vi "Autonomous Independent.vi"   [LabVIEW 2023]
doc: "This VI is called when autonomous begins, and will automatically be terminated when autonomous ends. You can carry out timed or sensor driven robot movement independently without needing to return to the caller."
uses:
  <vilib>/Rock Robotics/WPI/Utilities/WPI_GetSetVariantRefNum.vi
  <vilib>/Rock Robotics/WPI/RobotDrive/WPI_RobotDriveMecanumDrive_Cartesian.vi
  <vilib>/Rock Robotics/Network Tables/NT Read Number.vi
  <vilib>/Rock Robotics/Network Tables/NT Read String.vi
panel:
  # "Be sure to right-click and choose Data Operations>>Make Current Value default if you want to save the array values with the VI"
types:
  T1 = typedef "WPI_RobotDriveDevRef.ctl" = cluster{"DevStatus":errorcluster, "Motors[]":T2[], "Square Inputs":bool, "Max Output":dbl}
  T2 = typedef "WPI_MotorControlDeviceRef.ctl" = cluster{"DeviceStatus":errorcluster, "Type":T3, "PWM":cluster{"PWM Channel":T4, "DeadBand":T5}, "CAN":cluster{"Device Number":u8, "SetOutput VI Ref":variant, "GetOutput VI Ref":variant, "Enable VI Ref":variant, "Disable VI Ref":variant, "Data":variant}, "Invert":bool, "DIO PWM":cluster{"PWM \"Enable\" Channel":T4, "DIOChannel":T6, "PWM Rate":dbl}}
  T3 = typedef "WPI_MotorControlType.ctl" = enum16{"PWM", "CAN", "DIO PWM"}
  T4 = typedef "FPGA_DIOPWMChannel.ctl" = enum8{"PWM 0", "PWM 1", "PWM 2", "PWM 3", "PWM 4", "PWM 5", "PWM 6", "PWM 7", "PWM 8", "PWM 9", "PWM MXP 0", "PWM MXP 1", "PWM MXP 2", "PWM MXP 3", "PWM MXP 4", "PWM MXP 5", "PWM MXP 6", "PWM MXP 7", "PWM MXP 8", "PWM MXP 9", "Invalid"}
  T5 = typedef "WPI_PWMDeadband.ctl" = cluster{"Name":string, "maxPositivePwm":i32, "minPositivePwm":i32, "centerPwm":i32, "maxNegativePwm":i32, "minNegativePwm":i32, "angularRange":u16}
  T6 = typedef "FPGA_DIOChannel.ctl" = enum8{"DIO 0", "DIO 1", "DIO 2", "DIO 3", "DIO 4", "DIO 5", "DIO 6", "DIO 7", "DIO 8", "DIO 9", "DIO MXP 0", "DIO MXP 1", "DIO MXP 2", "DIO MXP 3", "DIO MXP 4", "DIO MXP 5", "DIO MXP 6", "DIO MXP 7", "DIO MXP 8", "DIO MXP 9", "DIO MXP 10", "DIO MXP 11", "DIO MXP 12", "DIO MXP 13", "DIO MXP 14", "DIO MXP 15", "SPI Port CS1", "SPI Port CS2", "SPI Port CS3", "SPI Port MISO", "SPI Port MOSI", "Invalid"}
  T7 = typedef "WPI_GyroDevRef.ctl" = cluster{"DevStatus":errorcluster, "Analog Channel":T8, "Gain (VoltsPerDegree/Second)":dbl, "Gyro Type":enum16{"Analog", "XRS450"}, "Handle":i32, "SPI Bus":T9, "Device Found":bool, "Sample Rate":dbl, "Calibrate On Open":bool, "Offset":dbl}
  T8 = typedef "FPGA_AIChannel.ctl" = enum8{"AI 0", "AI 1", "AI 2", "AI 3", "AI MXP 0", "AI MXP 1", "AI MXP 2", "AI MXP 3", "Invalid"}
  T9 = typedef "spi_bus.ctl" = enum16{"SPI On-Board, CS0", "SPI On-Board, CS1", "SPI On-Board, CS2", "SPI On-Board, CS3", "SPI MXP", "Invalid"}
  T10 = typedef "WPI_DigitalInputDevRef.ctl" = cluster{"DevStatus":errorcluster, "DIO Channel":T6}
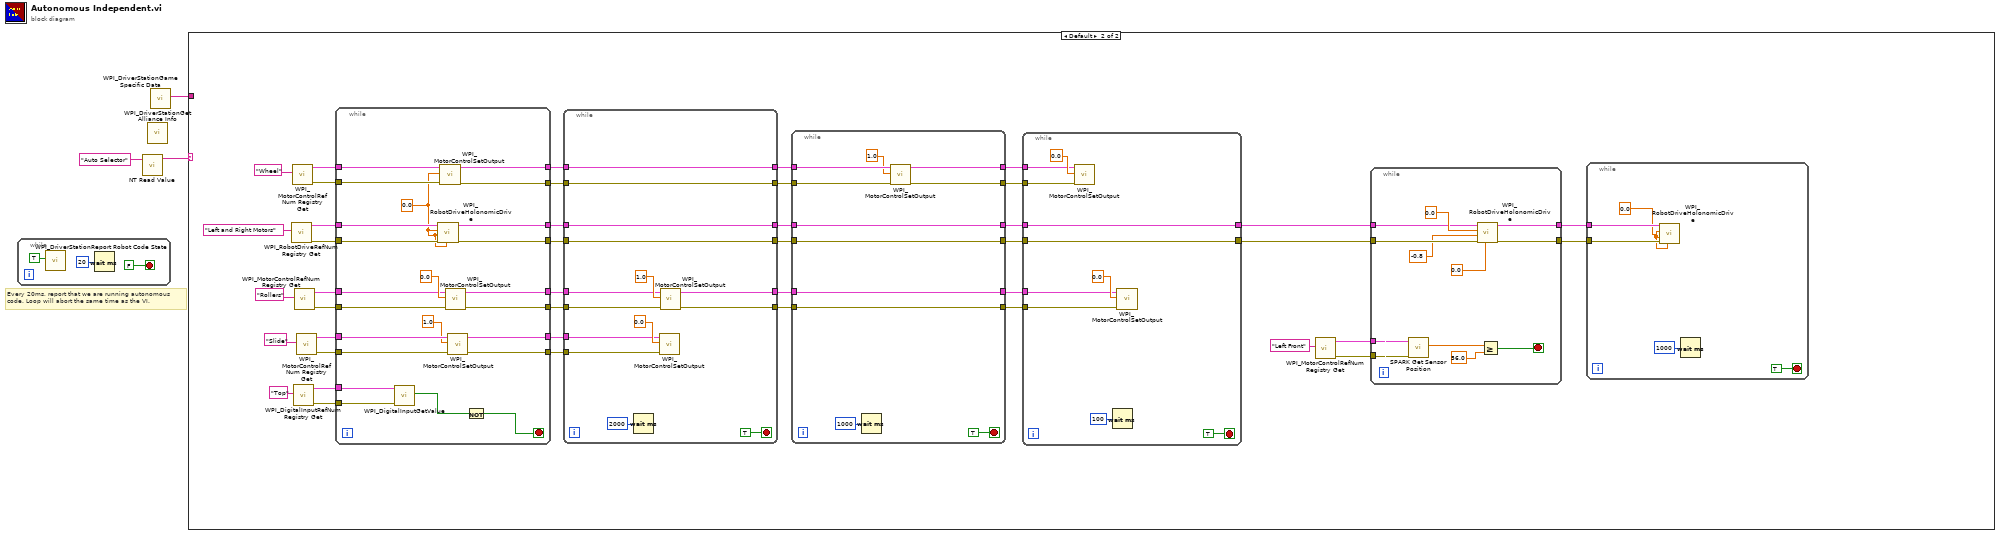
[diagram p0: block diagram]
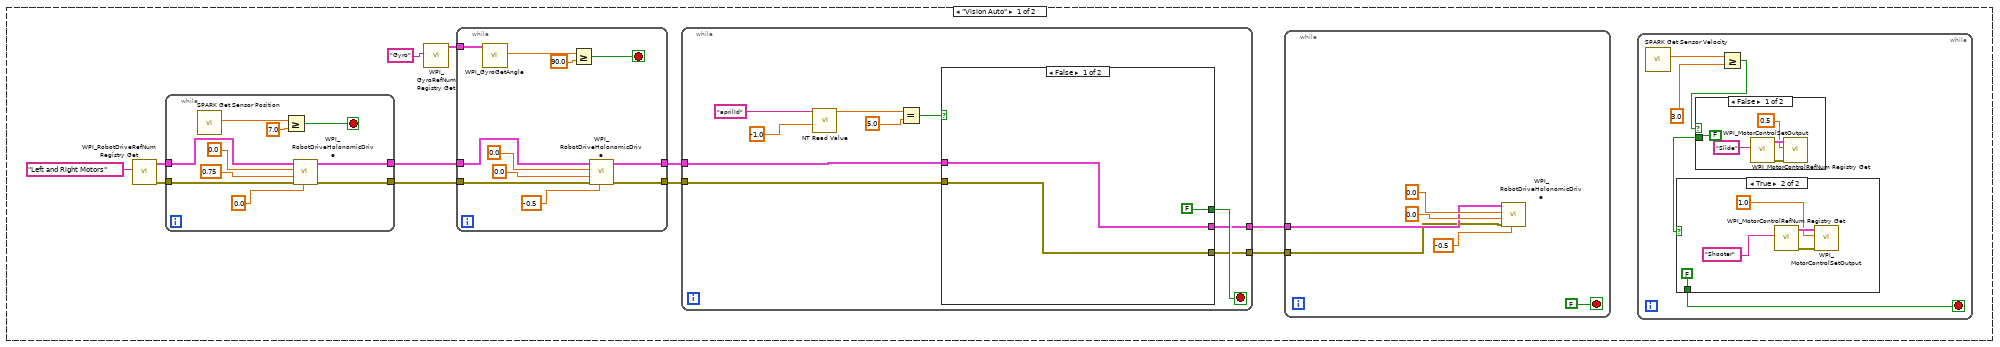
[diagram p2: hidden frame]
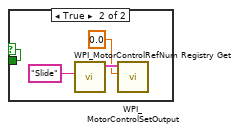
[diagram p3: hidden frame]
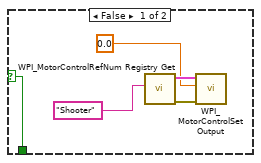
[diagram p4: hidden frame]
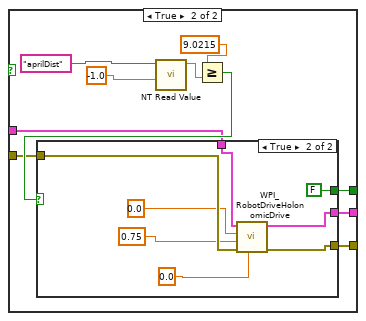
[diagram p5: hidden frame]
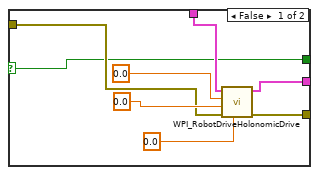
[diagram p6: hidden frame]
diagram:
  # "Every 20ms, report that we are running autonomous\ncode. Loop will abort the same time as the VI."
  n1 = while {
    stop <- FALSE stop-if-true
    n2 = call <vilib>:"WPI_DriverStationReport Robot Code State.vi"("Autonomous"=TRUE) -> ()  [unwired: 10 in, 1 out]
    n3 = Wait (ms)(milliseconds to wait=u32 20) -> ()  [unwired: 1 out]
  }
  n4 = call-poly <vilib>:"NT Read Value.vi"("name"="Auto Selector" ("Name")) -> ("value"=w2:string)  [unwired: 8 in, 2 out]
  n5 = call <vilib>:"WPI_DriverStationGet Alliance Info.vi"() -> ()  [unwired: 12 out]
  n6 = call <vilib>:"WPI_DriverStationGame Specific Data.vi"() -> ("Game Specific Data"=w1:string)  [unwired: 11 in]
  n7 = case shown="Default" w2 {
    tunnel: w1 -> [_ _]
    frame "Vision Auto" {
      n8 = call <vilib>:"WPI_RobotDriveRefNum Registry Get.vi"("refnum name"="Left and Right Motors") -> ("error out"=w16:errorcluster, "RobotDriveDevRef"=w15:T1)  [unwired: 1 in, 8 out]
      n9 = while {
        tunnel: w16 -> [w106]
        tunnel: w15 -> [w103]
        tunnel: [w99] -> w14
        tunnel: [w98] -> w13
        stop <- w100 stop-if-true
        n10 = call <vilib>:"SPARK Get Sensor Position.vi"() -> ("Sensor Position"=w102:dbl)  [unwired: 8 in, 3 out]
        n11 = Greater Or Equal?(x=w102, y=7.0) -> (x >= y?=w100:bool)
        n12 = call-poly <vilib>:"WPI_RobotDriveHolonomicDrive.vi"("Rotation"=0.0, "error in (no error)"=w106, "Y"=0.75, "X"=0.0, "RobotDriveDevRef"=w103) -> ("error out"=w98:errorcluster, "RobotDriveDevRef"=w99:T1)  [unwired: 4 in, 1 out]
      }
      n13 = call <vilib>:"WPI_GyroRefNum Registry Get.vi"("refnum name"="Gyro") -> ("GyroDevRef"=w11:T7)  [unwired: 9 in, 1 out]
      n14 = while {
        tunnel: w14 -> [w97]
        tunnel: w13 -> [w96]
        tunnel: w11 -> [w90]
        tunnel: [w88] -> w10
        tunnel: [w87] -> w9
        stop <- w89 stop-if-true
        n15 = call <vilib>:"WPI_GyroGetAngle.vi"("GyroDevRef"=w90) -> ("Angle"=w91:dbl)  [unwired: 6 in, 4 out]
        n16 = Greater Or Equal?(x=w91, y=90.0) -> (x >= y?=w89:bool)
        n17 = call-poly <vilib>:"WPI_RobotDriveHolonomicDrive.vi"("Rotation"=-0.5, "error in (no error)"=w96, "Y"=0.0, "X"=0.0, "RobotDriveDevRef"=w97) -> ("error out"=w87:errorcluster, "RobotDriveDevRef"=w88:T1)  [unwired: 4 in, 1 out]
      }
      n18 = while {
        tunnel: w10 -> [w51]
        tunnel: w9 -> [w52]
        tunnel: [w49] -> w8
        tunnel: [w48] -> w7
        stop <- w50 stop-if-true
        n19 = call-poly <vilib>:"NT Read Value.vi"("default value"=-1.0, "name"="aprilId") -> ("value"=w55:dbl)  [unwired: 7 in, 2 out]
        n20 = Equal?(x=w55, y=5.0) -> (x = y?=w53:bool)
        n21 = case shown="False" w53 {
          tunnel: w52 -> [w58 w65]
          tunnel: w51 -> [w59 w64]
          tunnel: [FALSE w63] -> w50
          tunnel: [w59 w62] -> w49
          tunnel: [w58 w61] -> w48
          frame False {
          }
          frame True {
            n22 = call-poly <vilib>:"NT Read Value.vi"("default value"=-1.0, "name"="aprilDist") -> ("value"=w70:dbl)  [unwired: 7 in, 2 out]
            n23 = Greater Or Equal?(x=9.0215, y=w70) -> (x >= y?=w66:bool)
            n24 = case shown="True" w66 {
              selector: w66 -> [w73 _]
              tunnel: w65 -> [w74 w85]
              tunnel: w64 -> [w75 w82]
              tunnel: [w73 FALSE] -> w63
              tunnel: [w72 w80] -> w62
              tunnel: [w71 w79] -> w61
              frame False {
                n25 = call-poly <vilib>:"WPI_RobotDriveHolonomicDrive.vi"("Rotation"=0.0, "error in (no error)"=w74, "Y"=0.0, "X"=0.0, "RobotDriveDevRef"=w75) -> ("error out"=w71:errorcluster, "RobotDriveDevRef"=w72:T1)  [unwired: 4 in, 1 out]
              }
              frame True {
                n26 = call-poly <vilib>:"WPI_RobotDriveHolonomicDrive.vi"("Rotation"=0.0, "error in (no error)"=w85, "Y"=0.75, "X"=0.0, "RobotDriveDevRef"=w82) -> ("error out"=w79:errorcluster, "RobotDriveDevRef"=w80:T1)  [unwired: 4 in, 1 out]
              }
            }
          }
        }
      }
      n27 = while {
        tunnel: w8 -> [w44]
        tunnel: w7 -> [w43]
        stop <- FALSE stop-if-true
        n28 = call-poly <vilib>:"WPI_RobotDriveHolonomicDrive.vi"("Rotation"=-0.5, "error in (no error)"=w43, "Y"=0.0, "X"=0.0, "RobotDriveDevRef"=w44) -> ()  [unwired: 4 in, 3 out]
      }
      n29 = while {
        stop <- w18 stop-if-true
        n30 = call <vilib>:"SPARK Get Sensor Velocity.vi"() -> ("Sensor Velocity"=w20:dbl)  [unwired: 8 in, 3 out]
        n31 = Greater Or Equal?(x=w20, y=3.0) -> (x >= y?=w21:bool)
        n32 = case shown="False" w21 {
          selector: w21 -> [_ w28]
          tunnel: [FALSE w28] -> w19
          frame False {
            n33 = call <vilib>:"WPI_MotorControlRefNum Registry Get.vi"("refnum name"="Slide") -> ("error out"=w26:errorcluster, "MotorControlDevRef"=w27:T2)  [unwired: 9 in]
            n34 = call <vilib>:"WPI_MotorControlSetOutput.vi"("error in (no error)"=w26, "Output"=0.5, "MotorControlDevRef"=w27) -> ()  [unwired: 6 in, 3 out]
          }
          frame True {
            n35 = call <vilib>:"WPI_MotorControlRefNum Registry Get.vi"("refnum name"="Slide") -> ("MotorControlDevRef"=w31:T2)  [unwired: 9 in, 1 out]
            n36 = call <vilib>:"WPI_MotorControlSetOutput.vi"("Output"=0.0, "MotorControlDevRef"=w31) -> ()  [unwired: 7 in, 3 out]
          }
        }
        n37 = case shown="True" w19 {
          selector: w19 -> [w32 _]
          tunnel: [w32 FALSE] -> w18
          frame False {
            n38 = call <vilib>:"WPI_MotorControlRefNum Registry Get.vi"("refnum name"="Shooter") -> ("error out"=w35:errorcluster, "MotorControlDevRef"=w36:T2)  [unwired: 9 in]
            n39 = call <vilib>:"WPI_MotorControlSetOutput.vi"("error in (no error)"=w35, "Output"=0.0, "MotorControlDevRef"=w36) -> ()  [unwired: 6 in, 3 out]
          }
          frame True {
            n40 = call <vilib>:"WPI_MotorControlRefNum Registry Get.vi"("refnum name"="Shooter") -> ("error out"=w40:errorcluster, "MotorControlDevRef"=w39:T2)  [unwired: 9 in]
            n41 = call <vilib>:"WPI_MotorControlSetOutput.vi"("error in (no error)"=w40, "Output"=1.0, "MotorControlDevRef"=w39) -> ()  [unwired: 6 in, 3 out]
          }
        }
      }
    }
    frame Default {
      n42 = call <vilib>:"WPI_RobotDriveRefNum Registry Get.vi"("refnum name"="Left and Right Motors") -> ("error out"=w137:errorcluster, "RobotDriveDevRef"=w138:T1)  [unwired: 1 in, 8 out]
      n43 = call <vilib>:"WPI_MotorControlRefNum Registry Get.vi"("refnum name"="Wheel") -> ("error out"=w120:errorcluster, "MotorControlDevRef"=w121:T2)  [unwired: 9 in]
      n44 = call <vilib>:"WPI_DigitalInputRefNum Registry Get.vi"("refnum name"="Top") -> ("error out"=w129:errorcluster, "DigitalInputDevRef"=w130:T10)  [unwired: 9 in]
      n45 = call <vilib>:"WPI_MotorControlRefNum Registry Get.vi"("refnum name"="Rollers") -> ("error out"=w141:errorcluster, "MotorControlDevRef"=w142:T2)  [unwired: 9 in]
      n46 = call <vilib>:"WPI_MotorControlRefNum Registry Get.vi"("refnum name"="Slide") -> ("error out"=w136:errorcluster, "MotorControlDevRef"=w135:T2)  [unwired: 9 in]
      n47 = while {
        tunnel: w142 -> [w192]
        tunnel: w141 -> [w191]
        tunnel: [w190] -> w140
        tunnel: [w189] -> w139
        tunnel: w138 -> [w188]
        tunnel: w137 -> [w187]
        tunnel: w135 -> [w185]
        tunnel: w136 -> [w186]
        tunnel: [w183] -> w133
        tunnel: [w182] -> w132
        tunnel: w130 -> [w181]
        tunnel: w129 -> [w180]
        tunnel: [w177] -> w128
        tunnel: [w176] -> w127
        tunnel: w121 -> [w175]
        tunnel: w120 -> [w174]
        tunnel: [w172] -> w119
        tunnel: [w171] -> w118
        stop <- w178 stop-if-true
        w173 = 0.0 ("X")
        n48 = call <vilib>:"WPI_DigitalInputGetValue.vi"("error in (no error)"=w180, "DigitalInputDevRef"=w181) -> ("Value"=w179:bool)  [unwired: 7 in, 2 out]
        n49 = call-poly <vilib>:"WPI_RobotDriveHolonomicDrive.vi"("Rotation"=w173, "error in (no error)"=w187, "Y"=w173, "X"=w173, "RobotDriveDevRef"=w188) -> ("error out"=w177:errorcluster, "RobotDriveDevRef"=w176:T1)  [unwired: 4 in, 1 out]
        n50 = call <vilib>:"WPI_MotorControlSetOutput.vi"("error in (no error)"=w174, "Output"=w173, "MotorControlDevRef"=w175) -> ("error out"=w171:errorcluster, "MotorControlDevRef"=w172:T2)  [unwired: 6 in, 1 out]
        n51 = call <vilib>:"WPI_MotorControlSetOutput.vi"("error in (no error)"=w191, "Output"=0.0, "MotorControlDevRef"=w192) -> ("error out"=w190:errorcluster, "MotorControlDevRef"=w189:T2)  [unwired: 6 in, 1 out]
        n52 = call <vilib>:"WPI_MotorControlSetOutput.vi"("error in (no error)"=w186, "Output"=1.0, "MotorControlDevRef"=w185) -> ("error out"=w182:errorcluster, "MotorControlDevRef"=w183:T2)  [unwired: 6 in, 1 out]
        n53 = Not(x=w179) -> (.not. x?=w178:bool)
      }
      n54 = while {
        tunnel: w140 -> [w206]
        tunnel: w139 -> [w205]
        tunnel: w133 -> [w203]
        tunnel: w132 -> [w202]
        tunnel: [w199] -> w125
        tunnel: w128 -> [w199]
        tunnel: [w198] -> w126
        tunnel: w127 -> [w198]
        tunnel: [w197] -> w124
        tunnel: [w196] -> w123
        tunnel: w119 -> [w195]
        tunnel: w118 -> [w194]
        tunnel: [w195] -> w117
        tunnel: [w194] -> w116
        stop <- TRUE stop-if-true
        n55 = Wait (ms)(milliseconds to wait=u32 2000) -> ()  [unwired: 1 out]
        n56 = call <vilib>:"WPI_MotorControlSetOutput.vi"("error in (no error)"=w202, "Output"=0.0, "MotorControlDevRef"=w203) -> ()  [unwired: 6 in, 3 out]
        n57 = call <vilib>:"WPI_MotorControlSetOutput.vi"("error in (no error)"=w206, "Output"=1.0, "MotorControlDevRef"=w205) -> ("error out"=w196:errorcluster, "MotorControlDevRef"=w197:T2)  [unwired: 6 in, 1 out]
      }
      n58 = while {
        tunnel: w123 -> [w162]
        tunnel: w124 -> [w163]
        tunnel: [w168] -> w112
        tunnel: w125 -> [w168]
        tunnel: [w167] -> w115
        tunnel: w126 -> [w167]
        tunnel: w117 -> [w166]
        tunnel: w116 -> [w165]
        tunnel: [w163] -> w111
        tunnel: [w162] -> w110
        tunnel: [w161] -> w109
        tunnel: [w160] -> w108
        stop <- TRUE stop-if-true
        n59 = Wait (ms)(milliseconds to wait=u32 1000) -> ()  [unwired: 1 out]
        n60 = call <vilib>:"WPI_MotorControlSetOutput.vi"("error in (no error)"=w165, "Output"=1.0, "MotorControlDevRef"=w166) -> ("error out"=w160:errorcluster, "MotorControlDevRef"=w161:T2)  [unwired: 6 in, 1 out]
      }
      n61 = while {
        tunnel: w115 -> [w157]
        tunnel: [w157] -> w114
        tunnel: [w156] -> w113
        tunnel: w112 -> [w156]
        tunnel: w111 -> [w155]
        tunnel: w110 -> [w154]
        tunnel: w109 -> [w153]
        tunnel: w108 -> [w152]
        stop <- TRUE stop-if-true
        n62 = call <vilib>:"WPI_MotorControlSetOutput.vi"("error in (no error)"=w152, "Output"=0.0, "MotorControlDevRef"=w153) -> ()  [unwired: 6 in, 3 out]
        n63 = Wait (ms)(milliseconds to wait=u32 100) -> ()  [unwired: 1 out]
        n64 = call <vilib>:"WPI_MotorControlSetOutput.vi"("error in (no error)"=w154, "Output"=0.0, "MotorControlDevRef"=w155) -> ()  [unwired: 6 in, 3 out]
      }
      n65 = call <vilib>:"WPI_MotorControlRefNum Registry Get.vi"("refnum name"="Left Front") -> ("error out"=w144:errorcluster, "MotorControlDevRef"=w143:T2)  [unwired: 9 in]
      n66 = while {
        tunnel: w113 -> [w223]
        tunnel: w114 -> [w220]
        tunnel: [w216] -> w147
        tunnel: [w215] -> w146
        tunnel: w143 -> [w214]
        tunnel: w144 -> [w213]
        stop <- w217 stop-if-true
        n67 = call <vilib>:"SPARK Get Sensor Position.vi"("error in (no error)"=w213, "MotorControlDevRef in"=w214) -> ("Sensor Position"=w219:dbl)  [unwired: 6 in, 3 out]
        n68 = call-poly <vilib>:"WPI_RobotDriveHolonomicDrive.vi"("Rotation"=0.0, "error in (no error)"=w223, "Y"=-0.8, "X"=0.0, "RobotDriveDevRef"=w220) -> ("error out"=w215:errorcluster, "RobotDriveDevRef"=w216:T1)  [unwired: 4 in, 1 out]
        n69 = Greater Or Equal?(x=w219, y=56.0) -> (x >= y?=w217:bool)
      }
      n70 = while {
        tunnel: w147 -> [w212]
        tunnel: w146 -> [w211]
        stop <- TRUE stop-if-true
        w210 = 0.0 ("Rotation")
        n71 = call-poly <vilib>:"WPI_RobotDriveHolonomicDrive.vi"("Rotation"=w210, "error in (no error)"=w211, "Y"=w210, "X"=w210, "RobotDriveDevRef"=w212) -> ()  [unwired: 4 in, 3 out]
        n72 = Wait (ms)(milliseconds to wait=u32 1000) -> ()  [unwired: 1 out]
      }
    }
  }
